vi "综合实验二.vi"() -> ()   [LabVIEW 2018]
uses:
  <vilib>/Math Plots/2D Math Plots/2D Compass/2D Compass XCtrl/2D Compass.xctl
  <vilib>/Math Plots/2D Math Plots/2D Compass/2D Compass Datatype/Public/Plot Helper (Vector).vi
  <vilib>/Math Plots/2D Math Plots/2D Compass/2D Compass Datatype/2D Compass Datatype.lvclass
panel:
  out "2D Compass 2":refnum<class "2D Plot Datatype.lvclass">[](xcontrol) caption="航行罗盘图"
  out "2D Compass 3":refnum<class "2D Plot Datatype.lvclass">[](xcontrol) caption="风力图"
  out "y":dbl
  in  "y值":dbl[](array[numeric])
  out "XY Graph":cluster{"Y":dbl[], "Y":dbl[]}[](graph) caption="运动轨迹图"
  in  "X值":dbl[](array[numeric])
  in  "轨迹刷新":bool
  out "X":dbl
  out "航速变化趋势图":dbl(graph)
  out "风力":dbl(knob) scale=0.0..10.0
  out "航速":dbl(knob) scale=0.0..20.0
  out "风力变化趋势图":dbl(graph)
  out "燃\n\n\n料":dbl(slide) scale=0.0..100.0
  out "风向":dbl(knob) scale=-180.0..180.0
  out "航向":dbl(knob) scale=-180.0..180.0
  in  "Y轴方向控制":dbl(knob) scale=-10.0..10.0
  in  "X轴方向控制":dbl(knob) scale=-10.0..10.0
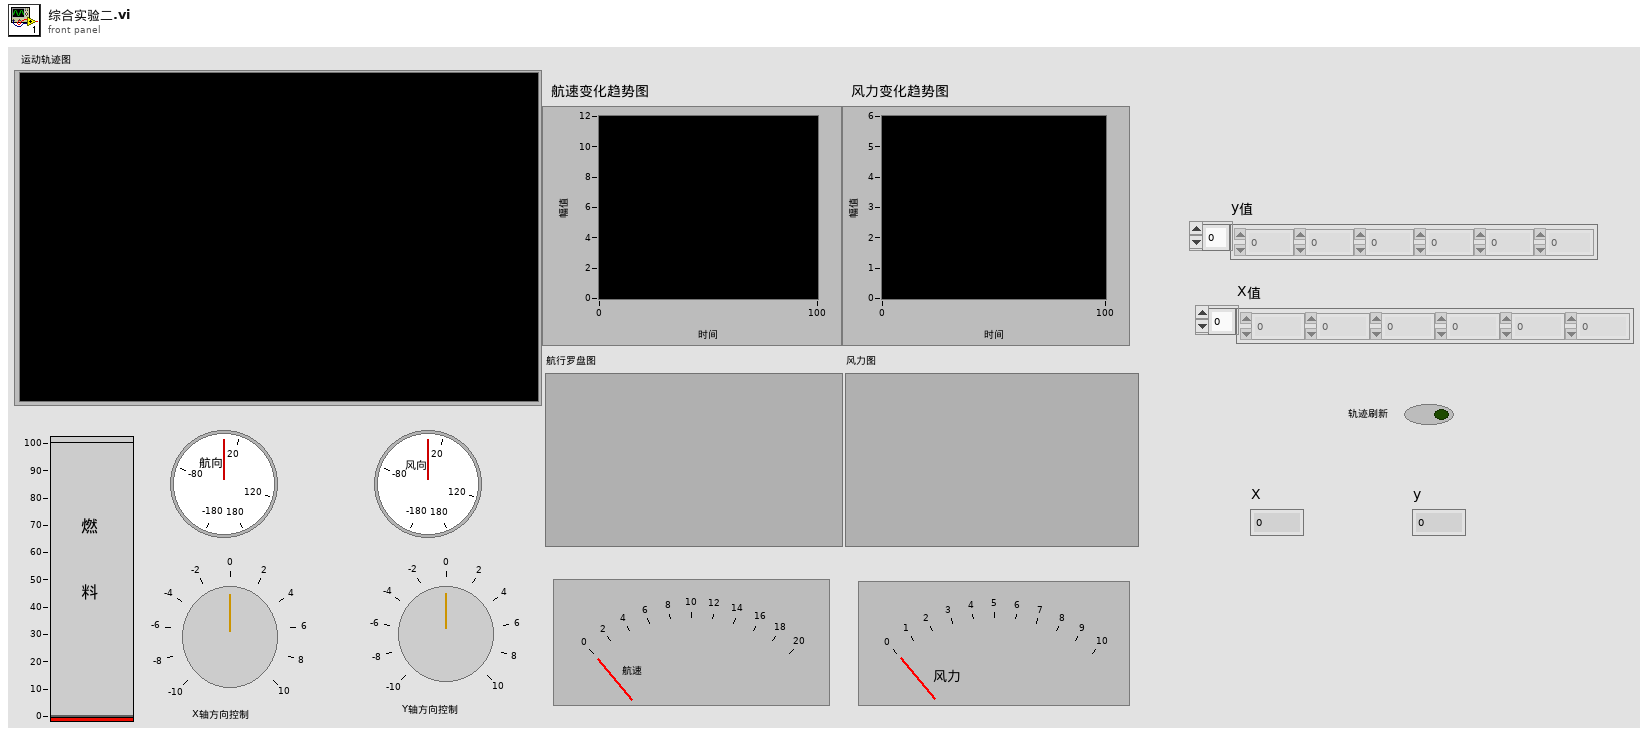
[diagram p1: front panel]
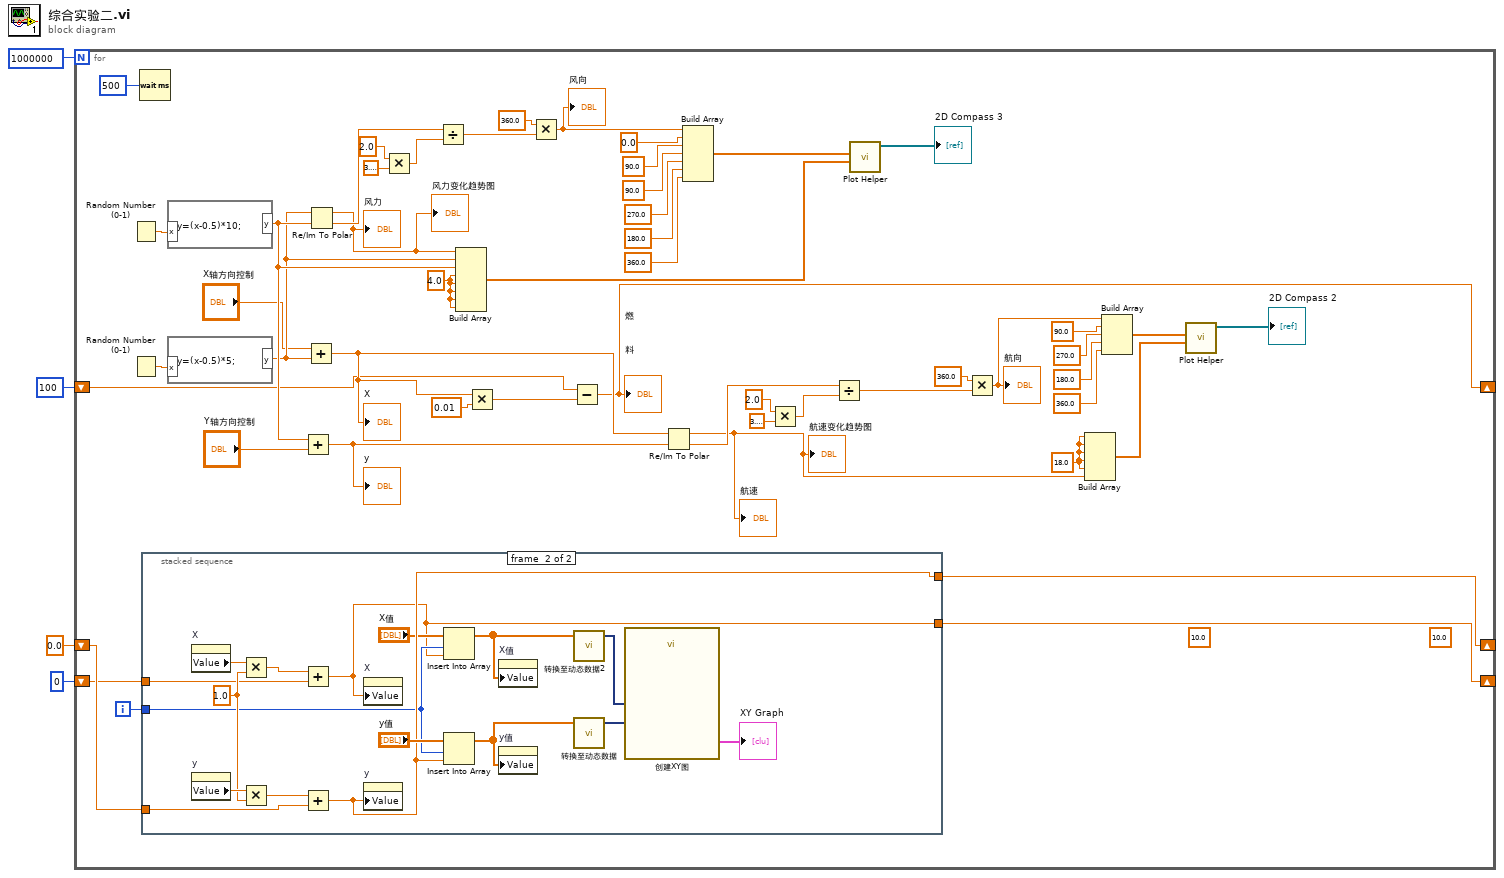
[diagram p0: block diagram]
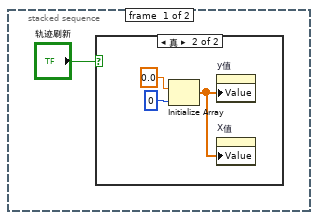
[diagram p2: hidden frame]
diagram:
  n1 = for {
    N: 1000000 -> [_]
    shift-right: [w20] -> _
    shift-left: 0.0 -> [w22]
    shift-right: [w19] -> _
    shift-left: 0 -> [w14]
    shift-right: [w9] -> _
    shift-left: 100 -> [w15]
    i -> [w21]
    w37 = 4.0 ("元素")
    w45 = 18.0 ("元素")
    (unwired) 10.0 ("x")
    (unwired) 10.0 ("x")
    n2 = Random Number (0-1)() -> (number: 0 to 1=w55:dbl)
    n3 = Random Number (0-1)() -> (number: 0 to 1=w54:dbl)
    n4 = Wait (ms)(milliseconds to wait=u32 500 ("等待时间（毫秒）")) -> ()  [unwired: 1 out]
    n5 = stacked-sequence {
      tunnel: w22 -> [_ w76]
      tunnel: w21 -> [_ w64]
      tunnel: [_ w71] -> w20
      tunnel: [_ w63] -> w19
      tunnel: w14 -> [_ w66]
      frame #0 {
        n6 = case shown="真" "轨迹刷新" {
          frame False {
          }
          frame True {
            n7 = Initialize Array(0.0 ("元素"), 0 ("维数大小")) -> (w58:dbl[])
            n8 = property on="y值" class="Arr (严格)"("Value"=w58) -> ()  [unwired: 2 in, 2 out]
            n9 = property on="X值" class="Arr (严格)"("Value"=w58) -> ()  [unwired: 2 in, 2 out]
          }
        }
      }
      frame #1 {
        w68 = 1.0 ("y")
        n10 = property on="X" class="DigNum (严格)"() -> ("Value"=w69:dbl)  [unwired: 2 in, 2 out]
        n11 = property on="y" class="DigNum (严格)"() -> ("Value"=w77:dbl)  [unwired: 2 in, 2 out]
        n12 = Multiply(x=w69, y=w68) -> (x*y=w67:dbl)
        n13 = Multiply(x=w77, y=w68) -> (x*y=w72:dbl)
        n14 = Add(x=w67, y=w66) -> (x+y=w63:dbl)
        n15 = Add(x=w72, y=w76) -> (x+y=w71:dbl)
        n16 = property on="X" class="DigNum (严格)"("Value"=w63) -> ()  [unwired: 2 in, 2 out]
        n17 = property on="y" class="DigNum (严格)"("Value"=w71) -> ()  [unwired: 2 in, 2 out]
        n18 = Insert Into Array(array="X值", index=w64, new element=w63) -> (w61:dbl[])
        n19 = Insert Into Array(array="y值", index=w64, new element=w71) -> (w70:dbl[])
        n20 = property on="X值" class="Arr (严格)"("Value"=w61) -> ()  [unwired: 2 in, 2 out]
        n21 = property on="y值" class="Arr (严格)"("Value"=w70) -> ()  [unwired: 2 in, 2 out]
        n22 = call "转换至动态数据2"("Array"=w61) -> ("Dynamic Data Type"=w62:dynamicdata)  [unwired: 3 in]
        n23 = call "转换至动态数据"("Array"=w70) -> ("Dynamic Data Type"=w73:dynamicdata)  [unwired: 3 in]
        n24 = call "创建XY图"("Y Input"=w73, "X Input"=w62) -> ("XY Graph"=→"XY Graph":cluster{"X":dbl[], "Y":dbl[]}[])  [unwired: 8 in, 1 out]
      }
    }
    n25 = formula code="y=(x-0.5)*10;"("x"=w55) -> ("y"=w24:dbl)
    n26 = formula code="y=(x-0.5)*5;"("x"=w54) -> ("y"=w23:dbl)
    n27 = Add(x=w24, y="Y轴方向控制") -> (x+y=w40:dbl)
    "y" <- w40
    n28 = Add(x="X轴方向控制", y=w23) -> (x+y=w16:dbl)
    "X" <- w16
    n29 = Re/Im To Polar(2:w24, 3:w23) -> (0:w25:dbl, 1:w10:dbl)
    "风力" <- w10
    "风力变化趋势图" <- w10
    n30 = Multiply(x=2.0, y=3.141592653589793) -> (x*y=w28:dbl)
    n31 = Divide(x=w25, y=w28) -> (x/y=w27:dbl)
    n32 = Build Array(w10, w23, w24, w37, w37, w37, w37, w37) -> (w38:dbl[])
    n33 = Multiply(x=w16, y=0.01) -> (x*y=w17:dbl)
    n34 = Multiply(x=360.0, y=w27) -> (x*y=w7:dbl)
    "风向" <- w7
    n35 = Subtract(x=w15, y=w17) -> (x-y=w9:dbl)
    "燃\n\n\n料" <- w9
    n36 = Re/Im To Polar(2:w40, 3:w16) -> (0:w47:dbl, 1:w11:dbl)
    "航速变化趋势图" <- w11
    "航速" <- w11
    n37 = Build Array(w7, 0.0 ("元素"), 90.0 ("元素"), 90.0 ("元素"), 270.0 ("元素"), 180.0 ("元素"), 360.0 ("元素")) -> (w13:dbl[])
    n38 = Multiply(x=2.0, y=3.141592653589793) -> (x*y=w50:dbl)
    n39 = Divide(x=w47, y=w50) -> (x/y=w49:dbl)
    n40 = call-poly <vilib>:"Plot Helper.vi"("radius vector"=w38, "theta vector"=w13) -> ("2D Plot Class Obj Array out"=→"2D Compass 3":refnum<class "2D Plot Datatype.lvclass">[])  [unwired: 2 in, 7 out]
    n41 = Multiply(x=360.0, y=w49) -> (x*y=w8:dbl)
    "航向" <- w8
    n42 = Build Array(w45, w45, w45, w45, w45, w11) -> (w12:dbl[])
    n43 = Build Array(w8, 90.0 ("元素"), 270.0 ("元素"), 180.0 ("元素"), 360.0 ("元素")) -> (w46:dbl[])
    n44 = call-poly <vilib>:"Plot Helper.vi"("radius vector"=w12, "theta vector"=w46) -> ("2D Plot Class Obj Array out"=→"2D Compass 2":refnum<class "2D Plot Datatype.lvclass">[])  [unwired: 2 in, 7 out]
  }
